vi "Test Y Interpolation.vi"() -> ()   [LabVIEW 2019]
uses:
  src/xy_utilities.lvlib
panel:
  in  "Fake Point":dbl
  out "Interpolated XY to 2D":dbl[][](graph)
  out "Interpolated XY":cluster{"X-array":dbl[], "Y-array":dbl[]}[](graph)
  out "XY Data":cluster{"X-array":dbl[], "Y-array":dbl[]}[](graph)
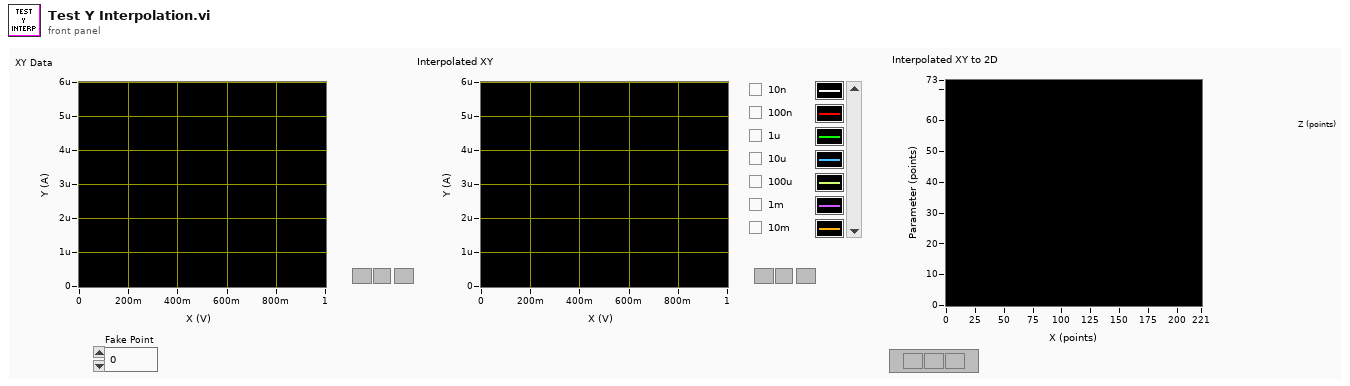
[diagram p1: front panel]
types:
  T1 = enum16{"thermal waveguide", "superlattice waveguide", "decay in atmosphere"}
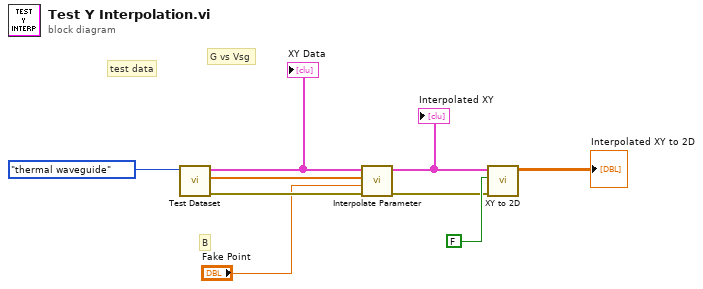
[diagram p0: block diagram]
diagram:
  # "B"
  # "G vs Vsg"
  # "test data"
  n1 = call "Test Dataset.vi"("Enum"=T1."thermal waveguide") -> ("error out"=w3:errorcluster, "Parameters out"=w6:dbl[], "XY-data out"=w9:cluster{"X-array":dbl[], "Y-array":dbl[]}[])  [unwired: 8 in]
  "XY Data" <- w9
  n2 = call "Interpolate Parameter.vi"("error in (no error)"=w3, "Fake Point"="Fake Point", "Parameter-array"=w6, "XY-data"=w9) -> ("error out"=w4:errorcluster, "Interpolated XY-data out"=w5:cluster{"X-array":dbl[], "Y-array":dbl[]}[])  [unwired: 5 in, 1 out]
  "Interpolated XY" <- w5
  n3 = call "XY to 2D.vi"("error in (no error)"=w4, "Interpolate [T]"=FALSE, "XY-data"=w5) -> ("2D Z Array"=→"Interpolated XY to 2D":dbl[][])  [unwired: 5 in, 3 out]
